vi "例程13-创建波形数据并获取其属性.vi"() -> ()   [LabVIEW 2016]
uses:
  <vilib>/measure/NI_MABase.lvlib
panel:
  out "波形图":waveform(dbl)(graph)
  out "类型":string
  out "数值":i32
  out "波形输出":waveform(dbl)
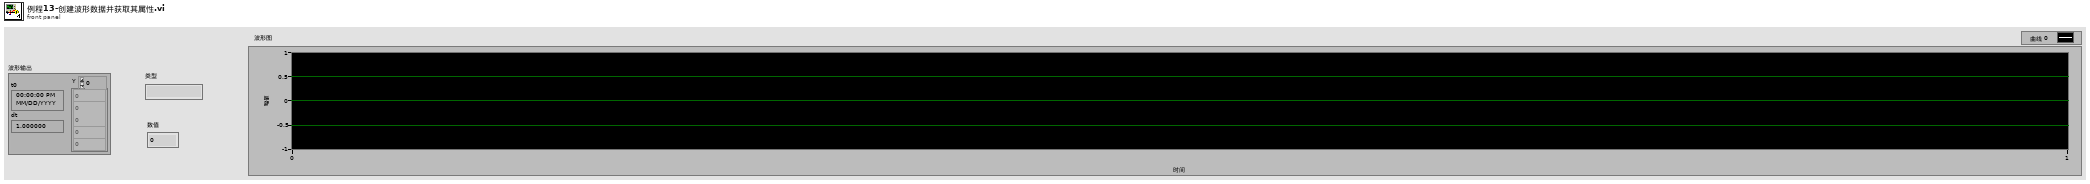
[diagram p1: front panel]
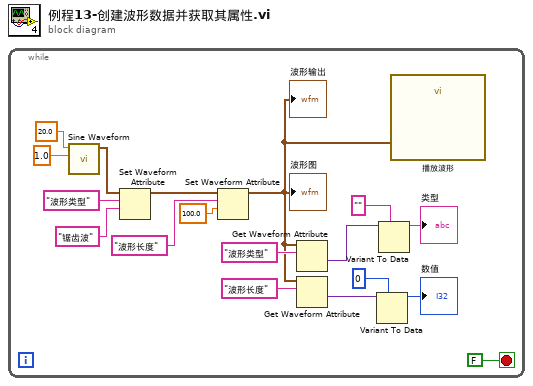
[diagram p0: block diagram]
diagram:
  n1 = while {
    stop <- FALSE stop-if-true
    n2 = call <vilib>:"Sine Waveform.vi"("amplitude"=1.0, "frequency"=20.0) -> ("signal out"=w16:waveform(dbl))  [unwired: 8 in, 1 out]
    n3 = Set Waveform Attribute(5:"锯齿波" ("名称"), 6:"波形类型" ("名称"), 7:w16) -> (3:w14:waveform(dbl))  [unwired: 1 in, 2 out]
    n4 = Set Waveform Attribute(5:100.0, 6:"波形长度" ("名称"), 7:w14) -> (3:w1:waveform(dbl))  [unwired: 1 in, 2 out]
    "波形输出" <- w1
    "波形图" <- w1
    n5 = Get Waveform Attribute(6:"波形类型" ("名称"), 7:w1) -> (1:w8:variant)  [unwired: 2 in, 3 out]
    n6 = Get Waveform Attribute(6:"波形长度" ("名称"), 7:w1) -> (1:w7:variant)  [unwired: 2 in, 3 out]
    n7 = Variant To Data(type=0, Variant=w7) -> (data=→"数值":i32)  [unwired: 1 in, 1 out]
    n8 = Variant To Data(type="" ("名称"), Variant=w8) -> (data=→"类型":string)  [unwired: 1 in, 1 out]
    n9 = call "播放波形"("Data"=w1) -> ()  [unwired: 18 in, 1 out]
  }
